vi "Parse Instrument.vi"(8 "error in (no error)":errorcluster, 10 "path to XML document":path=path "C:/Users/frmausse/Desktop/Summer Projects/VIStore (Actor)/Source/StoreCats.xml") -> (0 "error out":errorcluster, 3 "Instrument":refnum<class "Instrument.lvclass">)   [LabVIEW 2015, in "Item Actor.lvlib" / "Instrument.lvclass"]
uses:
  Instrument.lvclass
  Instrument.lvclass/Instrument.ctl
  Generic Item/Generic Item.lvclass/Generic Item.ctl
  Generic Item/Write Weight.vi
  <vilib>/xml/Load XML File.vi
  <vilib>/xml/Close Reference(Node).vi
  <vilib>/xml/NI_XML.lvlib
  <resource>/objmgr/DOMUserDefRef.rc
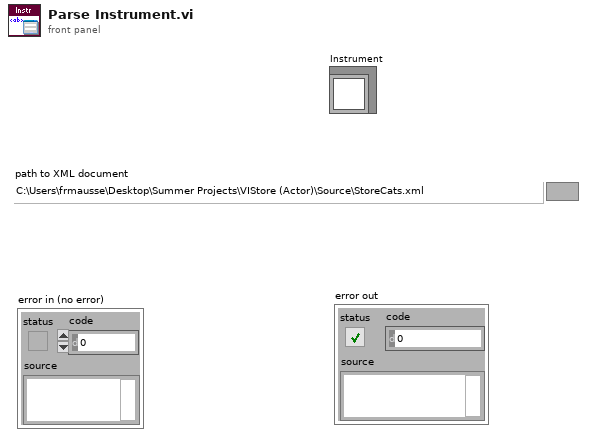
[diagram p1: front panel]
types:
  T1 = typedef "imagedata.ctl" = cluster{"image type":i32, "image depth":i32, "image":u8[], "mask":u8[], "colors":u32[], "Rectangle":cluster{"left":i16, "top":i16, "right":i16, "bottom":i16}}
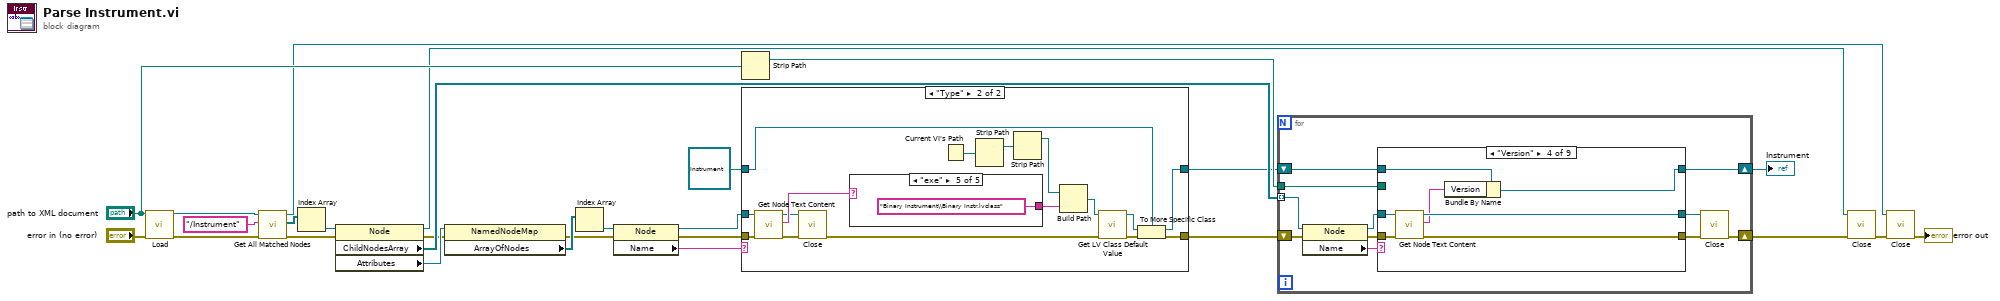
[diagram p0: block diagram]
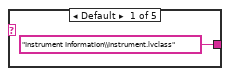
[diagram p3: hidden frame]
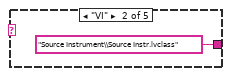
[diagram p4: hidden frame]
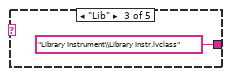
[diagram p5: hidden frame]
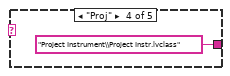
[diagram p6: hidden frame]
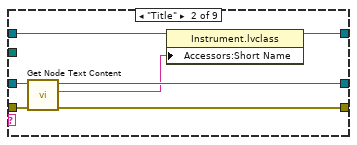
[diagram p8: hidden frame]
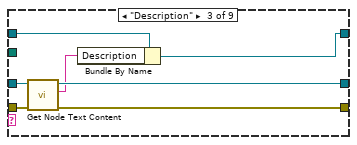
[diagram p9: hidden frame]
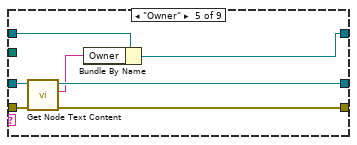
[diagram p10: hidden frame]
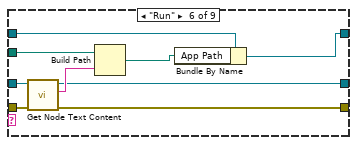
[diagram p11: hidden frame]
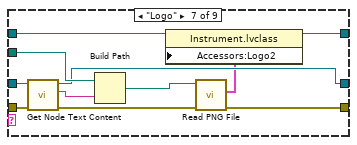
[diagram p12: hidden frame]
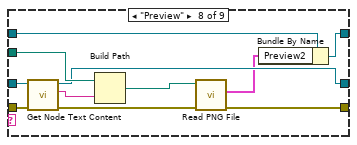
[diagram p13: hidden frame]
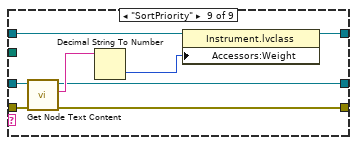
[diagram p14: hidden frame]
diagram:
  n1 = call-poly <vilib>:"Load.vi"("path to XML document"="path to XML document", "error in (no error)"="error in (no error)") -> ("DOM document out"=w23:refnum<k20>, "error out"=w24:errorcluster)  [unwired: 11 in, 1 out]
  n2 = call <vilib>:"Get All Matched Nodes.vi"("error in (no error)"=w24, "XPath expression"="/Instrument" ("Tag Name"), "node in"=w23) -> ("error out"=w20:errorcluster, "node result array"=w17:refnum<k20>[], "node out"=w21:refnum<k20>)  [unwired: 6 in]
  n3 = Index Array(array=w17) -> (element=w13:refnum<k20>)  [unwired: 1 in]
  n4 = property class="Node"(reference=w13, error in=w20) -> (reference out=w14:refnum<k20>, error out=w2:errorcluster, "ChildNodesArray"=w16:refnum<k20>[], "Attributes"=w11:refnum<k20>)
  n5 = property class="NamedNodeMap"(reference=w11, error in=w2) -> (error out=w5:errorcluster, "ArrayOfNodes"=w9:refnum<k20>[])  [unwired: 1 out]
  n6 = Index Array(array=w9) -> (element=w10:refnum<k20>)  [unwired: 1 in]
  n7 = property class="Node"(reference=w10, error in=w5) -> (reference out=w7:refnum<k20>, error out=w6:errorcluster, "Name"=w8:string)
  n8 = Strip Path(path="path to XML document") -> (stripped path=w26:path)  [unwired: 1 out]
  n9 = case shown="\"Type\"" w8 {
    tunnel: w7 -> [_ w45]
    tunnel: w6 -> [w28 w44]
    tunnel: [w28 w30] -> w1
    tunnel: refnum<class "Instrument.lvclass"> refnum ("Instrument Information.lvclass") -> [w29 w36]
    tunnel: [w29 w35] -> w3
    frame Default {
    }
    frame "Type" {
      n10 = call <vilib>:"Get Node Text Content.vi"("error in (no error)"=w44, "node in"=w45) -> ("error out"=w34:errorcluster, "node text"=w40:string, "node out"=w32:refnum<k20>)  [unwired: 7 in]
      n11 = call-poly <vilib>:"Close.vi"("error in (no error)"=w34, "node"=w32) -> ("error out"=w33:errorcluster)  [unwired: 7 in]
      n12 = case shown="\"exe\"" w40 {
        tunnel: ["Instrument Information\\Instrument.lvclass" "Source Instrument\\Source Instr.lvclass" "Library Instrument\\Library Instr.lvclass" "Project Instrument\\Project Instr.lvclass" "Binary Instrument\\Binary Instr.lvclass"] -> w39
        frame Default {
        }
        frame "VI" {
        }
        frame "Lib" {
        }
        frame "Proj" {
        }
        frame "exe" {
        }
      }
      n13 = Current VI's Path() -> (path=w43:path)
      n14 = Strip Path(path=w43) -> (stripped path=w42:path)  [unwired: 1 out]
      n15 = Strip Path(path=w42) -> (stripped path=w41:path)  [unwired: 1 out]
      n16 = Build Path(base path=w41, name or relative path=w39) -> (appended path=w38:path)
      n17 = call <vilib>:"Get LV Class Default Value.vi"("error in (no error)"=w33, "class path"=w38) -> ("error out"=w31:errorcluster, "object"=w37:refnum<class>)  [unwired: 8 in]
      n18 = To More Specific Class(target class=w36, reference=w37, error in=w31) -> (specific class reference=w35:refnum<class "Instrument.lvclass">, error out=w30:errorcluster)
    }
  }
  n19 = for {
    tunnel: w16 -> [w58] mode=indexing
    shift-right: [w60] -> w12
    shift-left: w3 -> [w61]
    tunnel: w26 -> [w59]
    shift-right: [w52] -> w15
    shift-left: w1 -> [w55]
    n20 = property class="Node"(reference=w58, error in=w55) -> (reference out=w57:refnum<k20>, error out=w56:errorcluster, "Name"=w54:string)
    n21 = case shown="\"Version\"" w54 {
      tunnel: w61 -> [w64 w67 w78 w85 w92 w101 w104 w123 w126]
      tunnel: [w64 w65 w77 w84 w91 w100 w103 w122 w125] -> w60
      tunnel: w59 -> [_ _ _ _ _ w99 w112 w121 _]
      tunnel: w57 -> [w63 w71 w76 w83 w90 w97 w111 w120 w131]
      tunnel: [w63 w70 w75 w82 w89 w95 w109 w118 w129] -> w51
      tunnel: [w62 w68 w73 w80 w87 w93 w106 w115 w128] -> w53
      tunnel: w56 -> [w62 w69 w74 w81 w88 w94 w108 w117 w127]
      frame Default {
      }
      frame "Title" {
        n22 = call <vilib>:"Get Node Text Content.vi"("error in (no error)"=w69, "node in"=w71) -> ("error out"=w68:errorcluster, "node text"=w66:string, "node out"=w70:refnum<k20>)  [unwired: 7 in]
        n23 = property class="Instrument.lvclass"(reference=w67, "Accessors:Short Name"=w66) -> (reference out=w65:refnum<class "Instrument.lvclass">)  [unwired: 1 in, 1 out]
      }
      frame "Description" {
        n24 = call <vilib>:"Get Node Text Content.vi"("error in (no error)"=w74, "node in"=w76) -> ("error out"=w73:errorcluster, "node text"=w72:string, "node out"=w75:refnum<k20>)  [unwired: 7 in]
        n25 = Bundle By Name(cluster=w78, "Description"=w72) -> (w77:refnum<class "Instrument.lvclass">)
      }
      frame "Version" {
        n26 = call <vilib>:"Get Node Text Content.vi"("error in (no error)"=w81, "node in"=w83) -> ("error out"=w80:errorcluster, "node text"=w79:string, "node out"=w82:refnum<k20>)  [unwired: 7 in]
        n27 = Bundle By Name(cluster=w85, "Version"=w79) -> (w84:refnum<class "Instrument.lvclass">)
      }
      frame "Owner" {
        n28 = call <vilib>:"Get Node Text Content.vi"("error in (no error)"=w88, "node in"=w90) -> ("error out"=w87:errorcluster, "node text"=w86:string, "node out"=w89:refnum<k20>)  [unwired: 7 in]
        n29 = Bundle By Name(cluster=w92, "Owner"=w86) -> (w91:refnum<class "Instrument.lvclass">)
      }
      frame "Run" {
        n30 = call <vilib>:"Get Node Text Content.vi"("error in (no error)"=w94, "node in"=w97) -> ("error out"=w93:errorcluster, "node text"=w96:string, "node out"=w95:refnum<k20>)  [unwired: 7 in]
        n31 = Build Path(base path=w99, name or relative path=w96) -> (appended path=w98:path)
        n32 = Bundle By Name(cluster=w101, "App Path"=w98) -> (w100:refnum<class "Instrument.lvclass">)
      }
      frame "Logo" {
        n33 = call <vilib>:"Get Node Text Content.vi"("error in (no error)"=w108, "node in"=w111) -> ("error out"=w107:errorcluster, "node text"=w110:string, "node out"=w109:refnum<k20>)  [unwired: 7 in]
        n34 = Build Path(base path=w112, name or relative path=w110) -> (appended path=w105:path)
        n35 = call <vilib>:"Read PNG File.vi"("error in (no error)"=w107, "path to PNG file"=w105) -> ("error out"=w106:errorcluster, "image data"=w102:T1)  [unwired: 7 in, 1 out]
        n36 = property class="Instrument.lvclass"(reference=w104, "Accessors:Logo2"=w102) -> (reference out=w103:refnum<class "Instrument.lvclass">)  [unwired: 1 in, 1 out]
      }
      frame "Preview" {
        n37 = call <vilib>:"Get Node Text Content.vi"("error in (no error)"=w117, "node in"=w120) -> ("error out"=w116:errorcluster, "node text"=w119:string, "node out"=w118:refnum<k20>)  [unwired: 7 in]
        n38 = Build Path(base path=w121, name or relative path=w119) -> (appended path=w114:path)
        n39 = call <vilib>:"Read PNG File.vi"("error in (no error)"=w116, "path to PNG file"=w114) -> ("error out"=w115:errorcluster, "image data"=w113:T1)  [unwired: 7 in, 1 out]
        n40 = Bundle By Name(cluster=w123, "Preview2"=w113) -> (w122:refnum<class "Instrument.lvclass">)
      }
      frame "SortPriority" {
        n41 = call <vilib>:"Get Node Text Content.vi"("error in (no error)"=w127, "node in"=w131) -> ("error out"=w128:errorcluster, "node text"=w130:string, "node out"=w129:refnum<k20>)  [unwired: 7 in]
        n42 = Decimal String To Number(string=w130) -> (number=w124:i32)  [unwired: 2 in, 1 out]
        n43 = property class="Instrument.lvclass"(reference=w126, "Accessors:Weight"=w124) -> (reference out=w125:refnum<class "Instrument.lvclass">)  [unwired: 1 in, 1 out]
      }
    }
    n44 = call-poly <vilib>:"Close.vi"("error in (no error)"=w53, "node"=w51) -> ("error out"=w52:errorcluster)  [unwired: 7 in]
  }
  "Instrument" <- w12
  n45 = call-poly <vilib>:"Close.vi"("error in (no error)"=w15, "node"=w14) -> ("error out"=w25:errorcluster)  [unwired: 7 in]
  n46 = call-poly <vilib>:"Close.vi"("error in (no error)"=w25, "node"=w21) -> ("error out"=→"error out":errorcluster)  [unwired: 7 in]
